vi "AlliGator Script Sum All Datasets in Folder.vi"(4 "Index Offsets (Default: None)":i32[](array[numeric]), 6 "Weights (Default: None)":dbl[](array[numeric]), 7 "Single File? (Default: False)":bool, 8 "Error In":errorcluster, 9 "AlliGator Data Series Type":T1, 10 "Path":path, 11 "Alligator Queue Elements in":T2[](array[typedef])) -> (0 "Error Out":errorcluster, 1 "Message":string, 2 "[Time-Series Path]":path[](array[path]), 3 "Alligator Queue Elements out":T2[](array[typedef]))   [LabVIEW 2021, in "AlliGator Accumulated Dataset.lvlib"]
doc: "Launches a series of steps loading each dataset in a series (including background correction) and adding them to a reset accumulated dataset. This script is followed by the usual series of steps after a new dataset is loaded (display, phasor plot update, phasor ratio or map overlay in image source and/or image ROI highlight in phasor plot)."
uses:
  AlliGator Accumulated Dataset.lvlib
  AlliGator Q Element.ctl
  AlliGator Q Event.ctl
  AlliGator Data Series Type.ctl
  AlliGator Variables List.ctl
  Alligator Elements Order in Action Stack.ctl
  AlliGator Settings List.ctl
  AlliGator Gate Arithmetic.ctl
  AlliGator Channel Arithmetic Action Parameters.ctl
  AlliGator Load Dataset Options.ctl
  AlliGator FLI Dataset Type.ctl
  AlliGator Add Action Array to Stack.vi
  <vilib>/Utility/error.llb/Error Cluster From Error Code.vi
  AlliGator Add Single Action to Stack.vi
  <vilib>/ErrorRing/Error Ring.xnode
  AlliGator Action Engine.lvlib
  AlliGator Globals, Variables & Constants.lvlib
  Strings/Strings.lvlib
  Files/Files.lvlib
  AlliGator Files.lvlib
  AlliGator Settings.lvlib
  AlliGator Dual-Channel Datasets.lvlib
panel:
  out "File Names":string[](array[string])
  out "# Time Points":i32
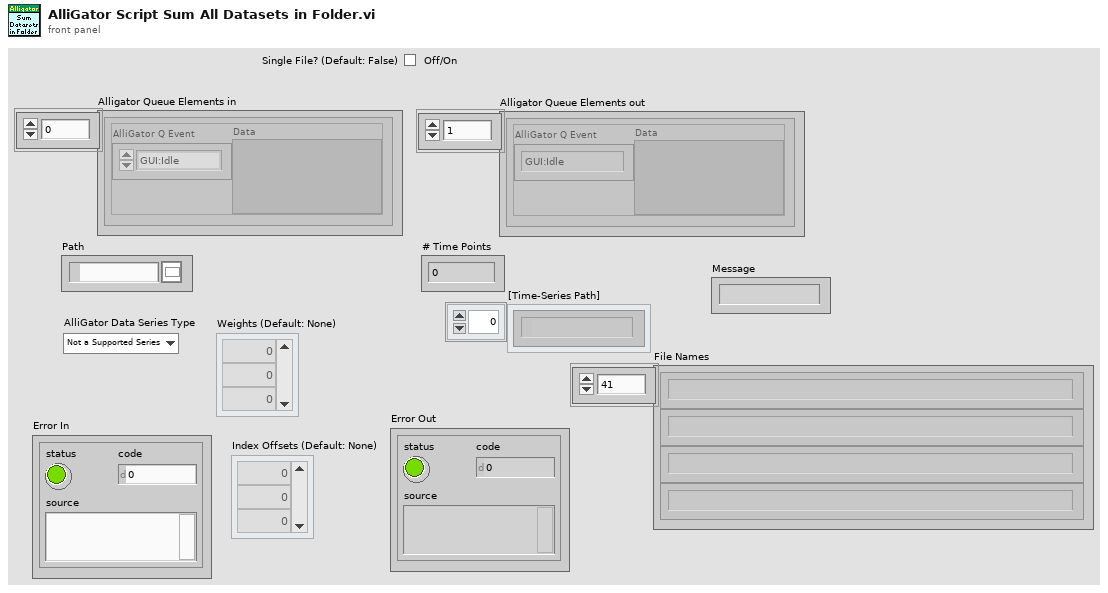
[diagram p1: front panel]
types:
  T1 = typedef "AlliGator Files.lvlib/AlliGator Data Series Type.ctl" = enum16{"Not a Supported Series", "Gate Images Folder Series", "SwissSPAD 2 Dataset Series", "B&H FLI Dataset Series", "PicoQuant PTU FLI Dataset Series", "PicoQuant BIN FLI Dataset Series", "Piccolo hist BIN FLI Dataset Series", "HDF5 FLI Dataset Series"}
  T2 = typedef "AlliGator Action Engine.lvlib/AlliGator Q Element.ctl" = cluster{"AlliGator Q Event":T3, "Data":variant}
  T3 = typedef "AlliGator Action Engine.lvlib/AlliGator Q Event.ctl" = enum16{"---- Files ----", "Files:Set Batch Export Files To Save", "Files:Set Dataset Loading & Pre-processing Options", "Files:Check #Frames in Dataset", "Files:Increment Frame Index", "Files:Open Mask Image", "Files:Open White Light Image", "Files:Open Single Dataset", "Files:New Folder of Folders Selected", "Files:Load File (all Types)_Scriptable", "Files:Move Flattened Series to Folders Series", "Files:Select Folder", "Files:Load FLI Dataset", "Files:Load Swiss SPAD 1 Dataset", "Files:Load Swiss SPAD 2 Dataset", "Files:Load .sdt FLI Dataset", "Files:Load .ptu FLI Dataset", "Files:Load .bin FLI Dataset", "Files:Load Single Gate Image Folder", "Files:Load I/m/phi Dataset (deprecated)", "Files:Load Single Image", "Files:Subtract Background File", "Files:Export FLI Dataset", "Files:Load HDF5 FLI Dataset", "Files:Set Destination File Path", "Files:Save Mask Image", "Files:Batch Conversion", "Files:New Folder Selected", "Files:Close FLI Dataset", "Files:Close FLI Dataset Series", "Files:Close White Light Image", "Files:Close Mask Image", "---- FLI Dataset ----", "FLI Dataset:Channel Arithmetic", "FLI Dataset:Export Average Lifetime Map as ASCII", "FLI Dataset:Export User-Defined Quantity Map as ASCII", "FLI Dataset:Python Function FLI Dataset Event", "FLI Dataset:ROI Analysis", "FLI Dataset:Tilted Logistic Square Gated IRF Characteristics Map", "FLI Dataset:Logistic Square Gated IRF Characteristics Map", "FLI Dataset:Square Gated IRF Characteristics Map", "FLI Dataset:Multi-ROI Single-Pixel Phasor Analysis", "FLI Dataset:Multi-ROI Single-Pixel NLSF Analysis", "FLI Dataset:All ROIs IRF Extraction", "FLI Dataset:All ROIs Decay Fit Non-Interactive (Fast + Individual IRF)", "FLI Dataset:All ROIs Phasor Analysis", "FLI Dataset:All ROIs Decay Fit", "FLI Dataset:Fluorescence Decay Statistics", "FLI Dataset:Update Decay Statistics Graph", "FLI Dataset:Get Decay from ROI", "FLI Dataset:All ROIs Average Lifetimes", "---- FLI Dataset Series ----", "FLI Dataset Series:Sum All Datasets in Series", "FLI Dataset Series:Add Dataset to Accumulated Dataset", "FLI Dataset Series:Display Accumulated Dataset", "FLI Dataset Series:Clear Dataset Series Sum", "FLI Dataset Series:Time-Series Analysis (NLSF)", "FLI Dataset Series:Time-Series Analysis (Phasor)", "---- Image ----", "Image:Update Image Profile Plots", "Image:Image Histogram Cursor Move", "Image:Image Histogram", "Image:Image Contrast", "Image:Set Image Histogram Cursor Move Flag", "Image:Clear Image Overlay", "Image:Use ROI as Search Area", "Image:Set ROI Diameter", "Image:Save Image Data as TIFF", "Image:Save Displayed Image with Overlay", "Image:Save Image Overlay Only", "Image:Save Image as Hot Pixel Mask", "Image:Change Source Image Color Palette", "Image:Copy Image to Clipboard", "Image:Source Image ROI Selection", "Image:Delete All ROIs", "Image:Delete All Unselected ROIs", "Image:Delete ROI", "Image:Merge All ROIs", "Image:Store ROI", "Image:Source Image ROI Storage", "Image:Export ROI Description to Notebook", "Image:Save ROI", "Image:Load ROI", "Image:Paste ROI Definition", "Image:Clear ROI", "Image:Identify ROIs in Mask Image", "Image:Create Complementary ROI", "Image:Create Contour ROI", "Image:Create ROI(s) from Pixels with Peak above Min_Scriptable", "Image:Create ROI(s) from Pixels with Intensity above Min_Scriptable", "Image:Compute ROI Statistics", "Image:Delete ROI(s) based on ROI Characteristics", "Image:Create ROI Grid", "Image:ROI to Individual Pixel ROIs", "Image:Python Function Source Image Event", "Image:Show Phasor Calibration Map ROI Centers", "Image:Convert ROI to Mask Image", "Image:Mouse Move", "Image:Mouse Up", "Image:Set Source Image Mouse Move Flag", "Image:Add Scale Bar Overlay", "Image:Delete Existing ROIs Option", "---- Decay ----", "Decay:Clear IRF/Reference Plot", "Decay:Clear Local IRFs", "Decay:Add Decay to Graph", "Decay:Smoothen Plot", "Decay:Smoothen Plot Tail", "Decay:Average Selected Plots", "Decay:Extract IRF", "Decay:Optimal IRF Extraction", "Decay:Threshold IRF", "Decay:Fit to Model IRF", "Decay:Fit IRF to Square Gate", "Decay:Fit IRF to Logistic Square Gate", "Decay:Fit IRF to Tilted Logistic Square Gate", "Decay:Create Bounding Cursors Set", "Decay:Export Bounding Cursors Definition to Notebook", "Decay:Denoise Plot", "Decay:Compute Cumulative Function", "Decay:Use as Reference Decay", "Decay:Show Reference Decay/IRF", "Decay:Extrapolate Decay", "Decay:Create Head & Tail Bounding Cursors", "Decay:Store Cursor-defined Head & Tail Fractions", "Decay:Rebin Plot", "Decay:1-Normalize Decay", "Decay:[0-1]-Normalize Plot", "Decay:Straighten Decay", "Decay:Shift Decay", "Decay:Fold Decay", "Decay:Fit Decay", "Decay:Global Fit of Selected Decays", "Decay:Post Global Fit Script", "Decay:Add Global Fit Parameters to Graph", "Decay:Add Decay Parameter(s) to Plot (Graph)", "Decay:Export Decay to Phasor Graph", "Decay:Plot Decay Shifts", "Decay:Compute Average Lifetime", "Decay:Plot Convolution", "Decay:Graph Tip Strip Update", "---- Decay Statistics ----", "Decay Statistics:Tip Strip Update", "---- Intensity Time Trace ----", "Intensity Time Trace:Use File Timestamp", "Intensity Time Trace:Load Intensity Corrections File", "Intensity Time Trace:Clear Intensity Corrections File", "Intensity Time Trace:Tip Strip Update", "---- Phasor Plot ----", "Phasor Plot:Build Phasor Plot", "Phasor Plot:Change Phasor Plot Color Palette", "Phasor Plot:Adjust Phasor Plot Display Range", "Phasor Plot:Highlight Image ROI in Phasor Plot", "Phasor Plot:Save Phasor Plot Image with Overlay", "Phasor Plot:Export Complex Phasor Map", "Phasor Plot:Export Phasor Ratio Map", "Phasor Plot:Export Average Lifetime Map", "Phasor Plot:Compute Phase Lifetime Histogram", "Phasor Plot:Compute Phasor Ratio Histogram", "Phasor Plot:Compute Phase Lifetime vs Intensity Scatter Plot", "Phasor Plot:Weber 2-Component Decomposition", "Phasor Plot:Update Phasor Color Map Vertices", "Phasor Plot:Clear Phasor Overlay", "Phasor Plot:Use Segment Extremities as References", "Phasor Plot:Use UC/Segment Intersections as References", "Phasor Plot:Use UC/Principal Axis Intersections as References", "Phasor Plot:Use UC/Linear Fit Intersections as References", "Phasor Plot:Update Phasor Plot Reference", "Phasor Plot:Show Local Phasor Info in Phasor Plot", "Phasor Plot:Update Phasor Plot State", "Phasor Plot:Phasor Plot ROI Storage", "Phasor Plot:Phasor Plot ROI Selection", "Phasor Plot:Python Function Phasor Plot Event", "Phasor Plot:Overlay Phasor ROI, Ratio or Map in Source Image", "Phasor Plot:Compute Decay of Selected Phasors", "Phasor Plot:Phasor at Image Pixel", "Phasor Plot:Mouse Move", "Phasor Plot:Mouse Up", "Phasor Plot:Display Range Mouse Move", "Phasor Plot:Set Mouse Move Flag", "---- Phasor Graph ----", "Phasor Graph:Calibrated Phasor Map Series", "Phasor Graph:Whole Image Phasor Scatter Plot (Todo)", "Phasor Graph:Get Phasor Value", "Phasor Graph:Create New Phasor Plot Dialog", "Phasor Graph:Update Last Phasor Value", "Phasor Graph:Update Phasor (m, phi)", "Phasor Graph:Remove Single Phasor from Plot", "Phasor Graph:Add Single Phasor to Plot", "Phasor Graph:Remove Phasor Plot", "Phasor Graph:Remove Selected Phasor Plots", "Phasor Graph:Clear Phasor Data", "Phasor Graph:Clear Phasor Graph", "Phasor Graph:Cursor Move", "Phasor Graph:Draw Cursor Connecting Line", "Phasor Graph:Clear Cursor Connecting Line", "Phasor Graph:Find UC Intersection", "Phasor Graph:Use UC/Cursor-Defined Line Intersections", "Phasor Graph:Use Selected Plots Fitted Line/UC Intersections", "Phasor Graph:Use Selected Plots Principal Axis/UC Intersections", "Phasor Graph:Show Single Phasor", "Phasor Graph:Save Single Phasor Plot", "Phasor Graph:Save All Phasor Plots", "Phasor Graph:Load Phasor Plot(s)", "Phasor Graph:Phasor Multiplication", "Phasor Graph:Compute Average Phasor", "Phasor Graph:Compute Multiple Average Phasors (Selected Plots)", "Phasor Graph:Export Single Phasor Plot Phase Lifetimes", "Phasor Graph:Phase Lifetime Trajectory", "Phasor Graph:Phase Lifetime vs Intensity Scatter Plot (deprecated)", "Phasor Graph:Parameter 2 vs Parameter 1 Scatter Plot", "Phasor Graph:Use Cursor n Location", "Phasor Graph:Set Reference n to Current Phase Lifetime Value", "Phasor Graph:Set Reference n to Lifetime Value", "Phasor Graph:Set Cursor n Location", "Phasor Graph:Save Phasor Graph Image", "Phasor Graph:Update SEPL Plot", "Phasor Graph:Export Single Phasor Plot Data", "Phasor Graph:Export Selected Phasor Plots Data", "Phasor Graph:Python Function Phasor Graph Event", "Phasor Graph:Tip Strip Update", "---- Calibration ----", "Calibration:Set Calibration Type", "Calibration:Load/Save Phasor Calibration", "Calibration:Load/Save Phasor Calibration Series", "Calibration:Load/Save Phasor Calibration Map", "Calibration:Use as Calibration", "Calibration:Compute Optimal Calibration from Phasor References", "Calibration:Clear Phasor Calibration", "Calibration:Use as Calibration Series", "Calibration:Use as Calibration Map", "Calibration:Clear Calibration Series", "Calibration:Clear Calibration Map", "Calibration:Apply Phasor Calibration", "Calibration:Update Single Plot Calibration", "Calibration:Update Multiple Plots Calibration", "Calibration:Clear Single Plot Calibration", "Calibration:Clear All Plots Calibrations", "Calibration:Clear Plot(s) Calibration(s)?", "Calibration:Phasor Calibration Maps (# Gates Series)", "---- Phasor Ratio ----", "Phasor Ratio:Clear Reference n", "Phasor Ratio:Toggle Selected Plot(s)  Lock to Reference 1", "Phasor Ratio:Use as Reference n", "Phasor Ratio:Send Reference n to Notebook", "Phasor Ratio:Toggle Selected Plot(s)  Lock to Reference 2", "Phasor Ratio:Compute Phasor Ratio at Mouse Location", "Phasor Ratio:Compute Phasor Plot's Average Phasor Ratio", "Phasor Ratio:Compute Time-Series Phasor Ratios", "Phasor Ratio:Fit Line to Phasor Ratio Plot", "Phasor Ratio:Save References", "Phasor Ratio:Load References", "Phasor Ratio:Update Phasor Reference 1", "Phasor Ratio:Update Phasor Reference 2", "Phasor Ratio:Move Cursor n to Reference n", "Phasor Ratio:Use as Phasor Reference 1 Lifetime", "Phasor Ratio:Use as Phasor Reference 2 Lifetime", "Phasor Ratio:Export Phasor Ratio Map as ASCII", "Phasor Ratio:Tip Strip Update", "---- Lifetime & Other Parameters Graph ----", "Lifetime:Tip Strip Update", "---- Decay Fit Parameter Map ----", "Decay Fit Parameter Map:Export ROI NLSF Data as ASCII", "Decay Fit Parameter Map:Set Decay Fit  Parameter Map Selection", "Decay Fit Parameter Map:Build Decay Fit Parameter Map", "Decay Fit Parameter Map:Change Decay Fit Parameter Map Color Palette", "Decay Fit Parameter Map:Export Decay Fit Parameter Map Data as ASCII", "Decay Fit Parameter Map:Export All Decay Fit Parameter Maps Data as ASCII", "Decay Fit Parameter Map:Send Map Data to Lifetime Graph", "Decay Fit Parameter Map:Save Decay Fit Parameter Map Image", "Decay Fit Parameter Map:Save-Load IRFs & Fit Data", "Decay Fit Parameter Map:Update Local Decay Plots", "Decay Fit Parameter Map:Python Function Decay Fit Parameters Map Event", "Decay Fit Parameter Map:Overlay Decay Fit Parameter Map in Source Image", "Decay Fit Parameter Map:Plot Map Data vs Intensity", "Decay Fit Parameter Map:Mouse Up", "Decay Fit Parameter Map:Display Range Mouse Move", "---- Generic Graph ----", "Generic Graph:Generic XY Graph Event", "Generic Graph:Python Function XY Graph Event", "Generic Graph:New Plot", "Generic Graph:Save Plot", "Generic Graph:XY Plot Histogram", "Generic Graph:Set XY Graph Plot Name", "Generic Graph:Set Last Cursor Style", "Generic Graph:Tip Strip Update", "---- GUI ----", "GUI:Start Script", "GUI:Type of Displayed Image Changed", "GUI:Gate Image Slide Changed", "GUI:Show Busy Icon", "GUI:Show Busy Icon & Abort Button", "GUI:Hide Busy Icon", "GUI:Hide Busy Icon & Abort Button", "GUI:Abort", "GUI:End Script", "GUI:Start Timing", "GUI:End Timing", "GUI:Set State Indicator", "GUI:Send Parameters JSON Strings to Clipboard", "GUI:Set Gate Step", "GUI:Idle", "GUI:Initialization", "GUI:Quit", "GUI:Increment Dataset Index", "GUI:Set Dataset Index to -1", "GUI:Time Series Slider Moved", "GUI:Time Series Slider Changed", "GUI:Toggle Playback or Loop", "GUI:Playback Script", "GUI:Set Phasor Frequency", "GUI:Open Window", "DEBUG"}
  T4 = typedef "AlliGator Globals, Variables & Constants.lvlib/AlliGator Variables List.ctl" = enum16{"---- GUI ----", "Initialization Status", "State Indicators Refnum", "Original AlliGator Menu Items", "Current Action Loop State", "Script in progress", "Playback", "Loop Playback", "Search ROI Used", "Search ROI", "Decay Graph Max Legend Size", "Intensity Graph Max Legend Size", "Decay Statistics Graph Max Legend Size", "Phasor Graph Max Legend Size", "Phasor Ratio Graph Max Legend Size", "Lifetime Graph Max Legend Size", "---- Files ----", "Export Dataset Frames as Individual Files", "Show Batch Export Help Balloons", "Frames in Dataset", "ptu File Frame Start Indices", "Current Frame in Dataset", "Current Frame Timestamp", "------ Python Plugins ------", "Python Plugins Information", "Python Session", "Valid Python Session?", "---- Source Image ----", "Dataset Loaded", "Dataset Metadata", "Dataset Channel", "Dataset Data Description", "Background Dataset Metadata", "Background Dataset Channel", "Background Dataset Data Description", "Background File Subtraction", "Background File Path", "Background File Pile-up Correction", "Background File Pixel Well Capacity", "Background File Scaling Factor", "Source Image ROIs", "Current Source Image ROI", "Source Image ROI Event Refnum", "X_Source Image Display Range", "X_Source Image Palette Information", "Source Image Palette List", "Source Image Scale", "Current Dataset Load Settings", "Source Image:ROI Overlay Color", "---- Image Profile Window ----", "Image Profile:Overlay ROI in Source Image", "Image Profile Window Event Refnum", "Image Profile:IntensityType", "Image Profile:Intensity Average Type", "Image Profile:Intensity-weighted SDV", "Image Profile:Box Profile Type", "Image Profile Window Open", "Image Profile:Plotted Fit Parameter", "X_Type of Displayed Image", "X_Time Gate Slider", "Dataset Path", "Source Image Overlay to Erase", "Is Displayed Image Accumulated", "White Light Image Modified", "Mask Image Modified", "Macrotime Gate Separation", "------ Phasor Graph -------", "Phasor Graph:Show Line", "---- Phasor Plot ---", "Phasor Plot Parameters Changed", "FLI Dataset Modified since last Phasor Plot Calculation", "Phasor Harmonics Data", "Selected Phasor Harmonics", "Phasor Harmonic Manager Event Refnum", "Phasor Plot ROIs", "Current Phasor Plot ROI", "Phasor Plot ROI Event Refnum", "Phasor Plot Image Reference Points", "Phasor Plot Computed", "Phasor Plot Palette Information", "Phasor Plot Palette List", "Phasor Ratio Palette Information", "Phasor Ratio Palette List", "Phasor Image Scale", "Phasor Plot Image Overlay to Erase", "Phasor Plot Image Elements to Update", "Current Phasor Plot Calculation Parameters", "Current Phasor Calibration Options", "Reset Cumulated Phasor Plot", "Phasor Ratio Reference 1", "Phasor Ratio Lifetime Reference 1", "Phasor Ratio Reference 1 Frequency", "Phasor Ratio Reference 2", "Phasor Ratio Lifetime Reference 2", "Phasor Ratio Reference 2 Frequency", "---- Decay Analysis ----", "Number of Selected Decays to Fit", "LS Fit Results", "LAR Fit Results", "BS Fit Results", "Last Decay Max - Min", "Best Fit Parameters", "Best Fit Parameter Names", "Actual Size X", "Actual Size Y", "Binning X", "Binning Y", "Actual # Gates", "Dataset Number", "Gates to...", "Gates Skipped", "Gates to keep", "Gate Step", "Gate Separation", "Reversed Gates", "Pile-up Correction", "Pixel Well Capacity", "Background Subtracted", "Background Subtraction Method", "Background Definition Range", "Background File (deprecated)", "Number of Dataset Accumulated", "Array of Accumulated Dataset Paths", "Do Averaged Datasets", "Destination File Path", "Process Plot Target", "Use 1/D as Phasor Frequency", "---- Decay Fit Parameter Map -----", "Decay Fit Parameter Map Palette Information", "Decay Fit Parameter Map Palette List", "Local Decay Graph Window Event Refnum", "------- Local Decay Window ---------", "Use normalized IRF for convolution", "----- Miscellaneous ----", "Skippable Dialog Windows Status"}
  T5 = enum16{"Start Script", "Load & Analyze Data", "End Script"}
  T6 = typedef "AlliGator Action Engine.lvlib/Alligator Elements Order in Action Stack.ctl" = enum16{"Enqueue 2 AFTER 1", "Enqueue 2 BEFORE 1"}
  T7 = typedef "AlliGator Dual-Channel Datasets.lvlib/AlliGator Channel Arithmetic Action Parameters.ctl" = cluster{"Channel Name":u16, "Channel Arithmetic":T8}
  T8 = typedef "AlliGator Settings.lvlib/AlliGator Gate Arithmetic.ctl" = enum16{"None", "INT-G2", "G2/INT*<INT>", "(1 - G2/INT)*<INT>"}
  T9 = typedef "AlliGator Settings.lvlib/AlliGator Settings List.ctl" = enum16{"GUI:Visible Settings Tab", "GUI:Last Run Version", "Source Image:Use Image Histogram for Contrast", "Source Image:Low Count Pixels Rejection Options", "Source Image:High Count Pixels Rejection Options", "Source Image:Use Image Brightness", "Source Image:Blend Overlay with Image Background", "Source Image:Use Fixed ROI Diameter", "Source Image:ROI Diameter", "Source Image:ROI Center Color", "Source Image:Peak Threshold", "Source Image:Intensity Threshold", "Source Image:Image Binning Options", "Source Image:Image Smoothing Options", "Source Image:Image Histogram Active", "Source Image:Invert Binary Mask", "Source Image:Hot Pixel Removal", "Source Image:Overlay Analyzed ROI Center", "Source Image:Auto-Adjust Contrast", "Source Image:Histogram Lower Percentile", "Source Image:Histogram Upper Percentile", "Source Image:Save Source Image", "Source Image:Scale Bar Options", "Source Image:Image Resolution (Pixel Size)", "Source Image:Flatfield Correction", "Data Information:Gate Width", "Data Information:Nanotime Gate Separation", "Data Information:Macrotime Gate Separation", "Data Information:Gate Step", "Data Information:# Gates", "Data Information:Gate Image Exposure", "Data Information:Gate Image Integration", "Data Information:Gates to Skip", "Data Information:Gates to Keep", "Data Information:Define Gates to", "Data Information:Channel Name", "Data Information:Available Channel Names", "Data Information:Channel Arithmetic", "Data Information:Background File Subtraction", "Data Information:Background File", "Data Information:Background Scaling Factor", "Data Information:Background Pile-up Correction", "Data Information:Background Pixel Well Capacity", "Data Information:Laser Period", "Data Information:SYNC Period", "Data Information:Pile-up Correction", "Data Information:Pixel Well Capacity", "Data Information:Dataset Scaling Factor", "Fluorescence Decay_Decay Pre-Processing:Reverse Gates", "Fluorescence Decay_Decay Pre-Processing:Verbose Decay Pre-Processing", "Fluorescence Decay_Decay Pre-Processing:Use Decay Pre-Processing", "Fluorescence Decay_Decay Pre-Processing:Background Subtraction", "Fluorescence Decay_Decay Pre-Processing:Background Definition Range", "Fluorescence Decay_Decay Pre-Processing:Baseline Subtraction Method", "Fluorescence Decay_Decay Pre-Processing:Operations Order", "Fluorescence Decay_Decay Pre-Processing:Smoothing Parameter", "Fluorescence Decay_Decay Pre-Processing:Shift Decay", "Fluorescence Decay_Decay Pre-Processing:Decay Shift Parameters", "Fluorescence Decay_Decay Pre-Processing:Fold Decay", "Fluorescence Decay_Decay Pre-Processing:# Folds", "Fluorescence Decay_Decay Pre-Processing:1-Normalize Decay", "Fluorescence Decay_Decay Pre-Processing:[0-1]-Normalize Decay", "Fluorescence Decay_Decay Pre-Processing:Smoothen Decay", "Fluorescence Decay_Decay Pre-Processing:Extrapolate Decay", "Fluorescence Decay_Decay Pre-Processing:Use Periodicity", "Fluorescence Decay_Decay Pre-Processing:Use Cursors", "Fluorescence Decay_Decay Pre-Processing:Tail Fraction", "Fluorescence Decay_Decay Pre-Processing:Head Fraction", "Fluorescence Decay_Decay Pre-Processing:Additional Points", "Fluorescence Decay_Decay Pre-Processing:Straighten Decay", "Fluorescence Decay_Decay Pre-Processing:Constant Background", "Fluorescence Decay_Decay Pre-Processing:Pixel-Normalize Decay", "Fluorescence Decay_Advanced Analysis:Extract IRF instead of Decay", "Fluorescence Decay_Advanced Analysis:IRF Extraction Options", "Fluorescence Decay_Advanced Analysis:IRF Optimization Options", "Fluorescence Decay_Advanced Analysis:Square Pulse Options", "Fluorescence Decay_Advanced Analysis:IRF Order", "Fluorescence Decay_Advanced Analysis:IRF Time Constants", "Fluorescence Decay_Advanced Analysis:Wavelet Analysis Options", "Fluorescence Decay_Advanced Analysis:Average Lifetime Options", "Fluorescence Decay_Fit Options:Fit Options", "Fluorescence Decay_Fit Options:Use Legacy Fitting Approach", "Fluorescence Decay_Fit Options:Use Data Information Laser Period", "Fluorescence Decay_Fit Parameters:Displayed Fit Parameters", "Fluorescence Decay_Fit Parameters:Fit Parameter Constraints", "Fluorescence Decay_Fit Parameters:Export Tabulated Results", "Fluorescence Decay_Fit Parameters:MLE Baseline Offset Type", "Fluorescence Decay_Fit Parameters:MLE Baseline Offset", "Fluorescence Decay_Fit Parameters:Guess Parameter Names", "Fluorescence Decay_Fit Parameters:Guess Parameter Values", "Fluorescence Decay_Fit Parameters:Guess Parameters Options", "Fluorescence Decay_Styles:Show Last Decay Only", "Fluorescence Decay_Styles:Decay Graph Color Array", "Fluorescence Decay:Decay Graph Active", "Fluorescence Decay Statistics:Min Peak Value", "Fluorescence Decay Statistics:Reject Low Decay Peak Pixels", "Fluorescence Decay Statistics:Reject High Decay Peak Pixels", "Fluorescence Decay Statistics:Max Peak Value", "Time Traces:Use File Timestamp", "Time Traces:Time Step", "Time Traces:Use Intensity Correction File", "Time Traces:Intensity Correction File", "Phasor Plot:Phasor Plot Smoothing Options", "Phasor Plot:Phasor Plot Size", "Phasor Plot:Phasor Plot Graphics Options", "Phasor Plot:Cumulative Phasor Plot", "Phasor Plot:Use Phasor Brightness", "Phasor Plot:Blend Overlay with Phasor Background", "Phasor Plot:Save Phasor Plot", "Phasor Plot:Show References", "Phasor Plot:Phasor Ratio Decay Range", "Phasor Plot:Exponential Fading", "Phasor Plot:Phasor Ratio Reference Colors", "Phasor Plot:Reference Radius", "Phasor Plot:Show Color Map Vertices", "Phasor Plot:Phasor Plot Active", "Phasor Plot:Phasor Ratio Color Map Type", "Phasor Plot:Phasor Ratio Color Map", "Phasor Plot:Phasor Ratio Display Range", "Phasor Plot:Selected Image ROI(s)", "Phasor Plot:All Image ROIs", "Phasor Plot:Selected Phasor Plot ROI(s)", "Phasor Plot:All Phasor Plot ROIs", "Phasor Plot:Phasor Ratio Color-Coded Quantity", "Phasor Plot:Store Phasor Harmonics", "Phasor Plot:Draw Reference Segment", "Phasor Plot:User-Defined Quantity", "Phasor Graph:Phasor Frequency", "Phasor Graph:Phasor Ratio Type", "Phasor Graph:Pixel-level Phasor Computation", "Phasor Graph:Save Phasor Graph", "Phasor Graph:Phasor Graph Active", "Phasor Graph:Phasor SDV Options", "Phasor Calibration:Use Backup Calibration if needed", "Phasor Graph:Define Shortest Lifetime as", "Phasor Calibration:Backup Calibration Type", "Phasor Calibration:Calibration Type", "Phasor Calibration:Calibration Lifetime", "Phasor Calibration:Calibration Map Algorithm", "Single-Exponential Phasor Locus (SEPL):Gate Parameters", "Single-Exponential Phasor Locus (SEPL):User-defined Gate", "Single-Exponential Phasor Locus (SEPL):User-defined IRF", "Single-Exponential Phasor Locus (SEPL):Phasor Parameters", "Single-Exponential Phasor Locus (SEPL):Decay & IRF Parameters", "Single-Exponential Phasor Locus (SEPL):Display Parameters", "Lifetime Analysis:Decay Analysis Parameters", "Lifetime Analysis:Lifetime Map Active", "Plugins:Python Settings", "Miscellaneous:Verbose Mode", "Miscellaneous:Beep after Script", "Miscellaneous:Saved Image File Format", "Miscellaneous:Exported Gate Image Settings", "Miscellaneous:Include Loading in Timing", "Miscellaneous:Verbose Settings Mode", "Miscellaneous:Histogram Options", "Miscellaneous:Beep on Error", "Miscellaneous:# Logical Processors Used", "Miscellaneous:ROI Description Max Characters", "Miscellaneous:Verbose Error Mode", "Miscellaneous:Transparent Mask Color"}
  T10 = typedef "AlliGator Files.lvlib/AlliGator FLI Dataset Type.ctl" = enum16{"HDF5 FLI Dataset", "Gate Image Folder", ".sdt FLI Dataset (Becker & Hickl)", ".ptu FLI Dataset (PicoQuant)", "SS1 FLI Dataset", "SS2 FLI Dataset", "I/m/phi Dataset", ".bin FLI Dataset (PicoQuant Binned)", ".bin FLI Dataset (Piccolo Binned)"}
  T11 = typedef "AlliGator Files.lvlib/AlliGator Load Dataset Options.ctl" = cluster{"FLI Dataset Type":T10, "No Dialog?":bool, "File Path":path}
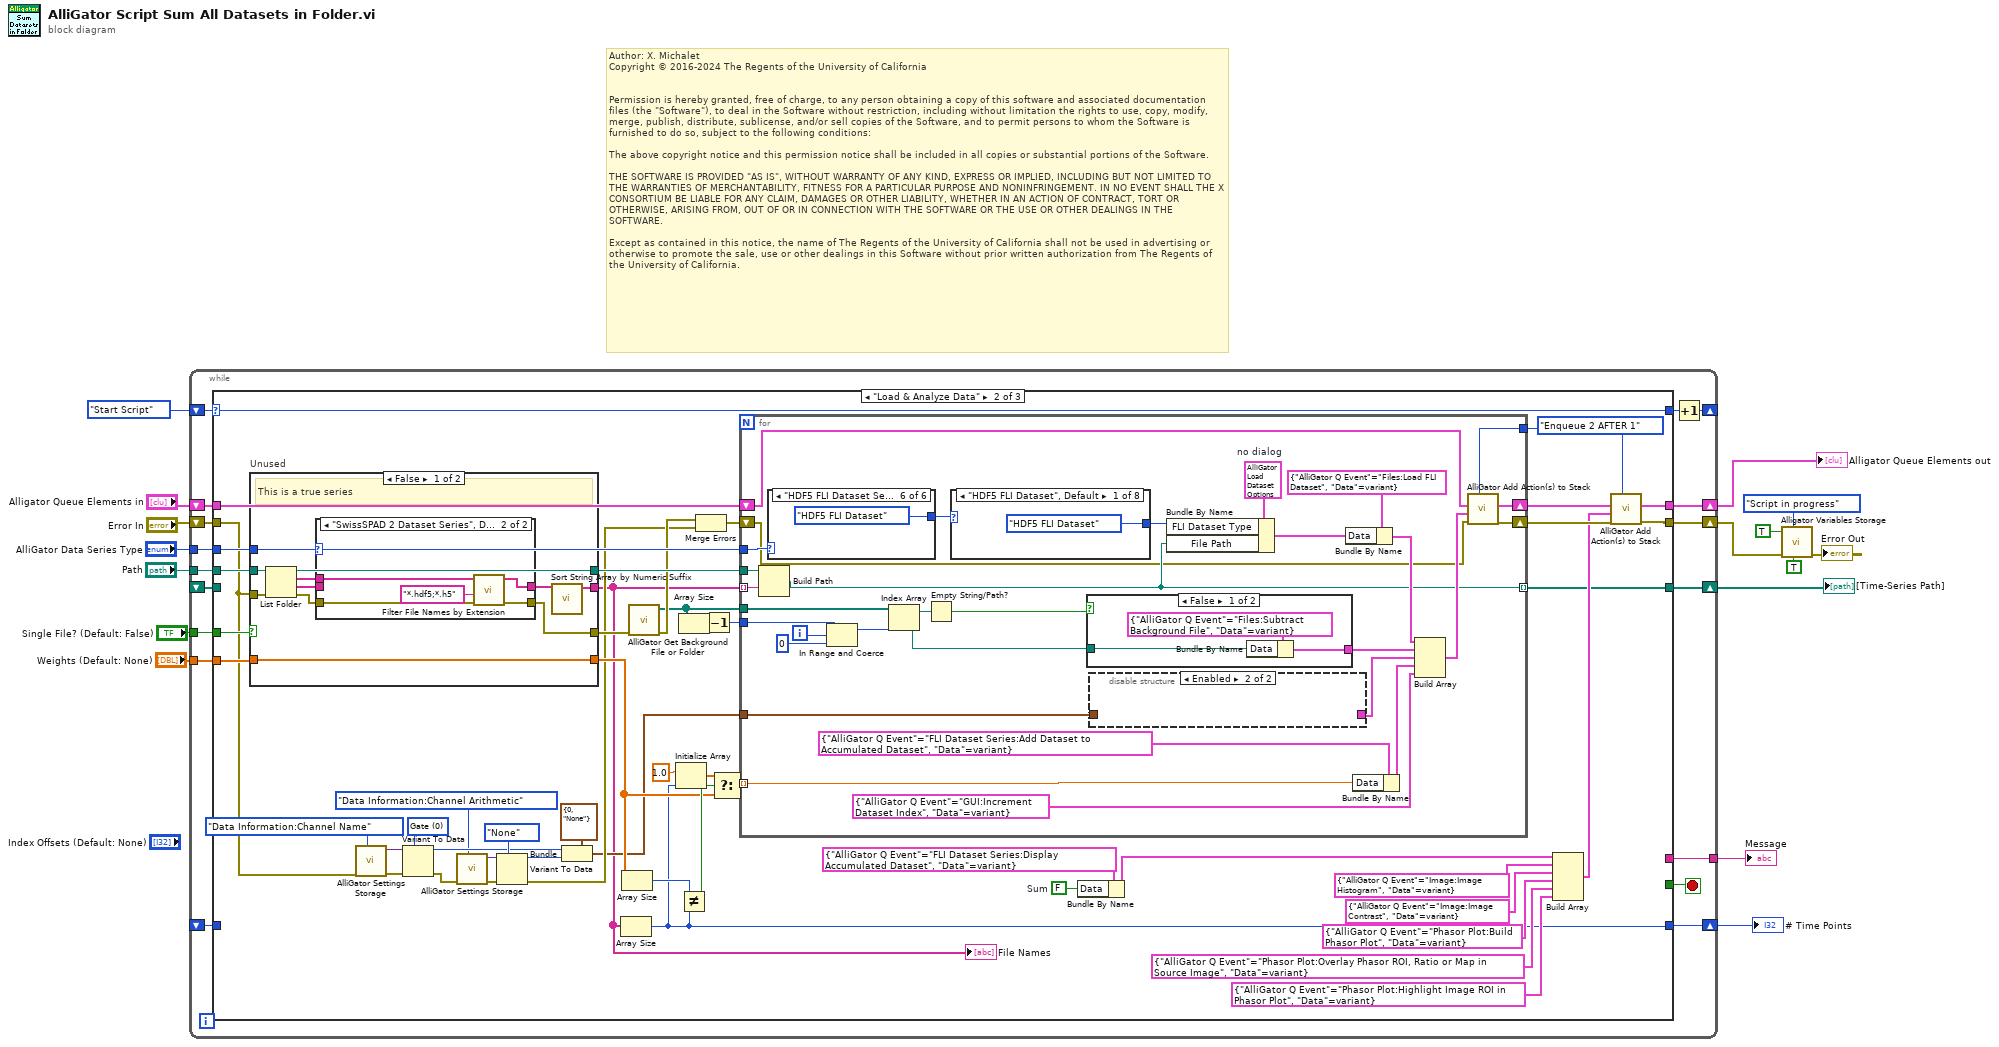
[diagram p0: block diagram]
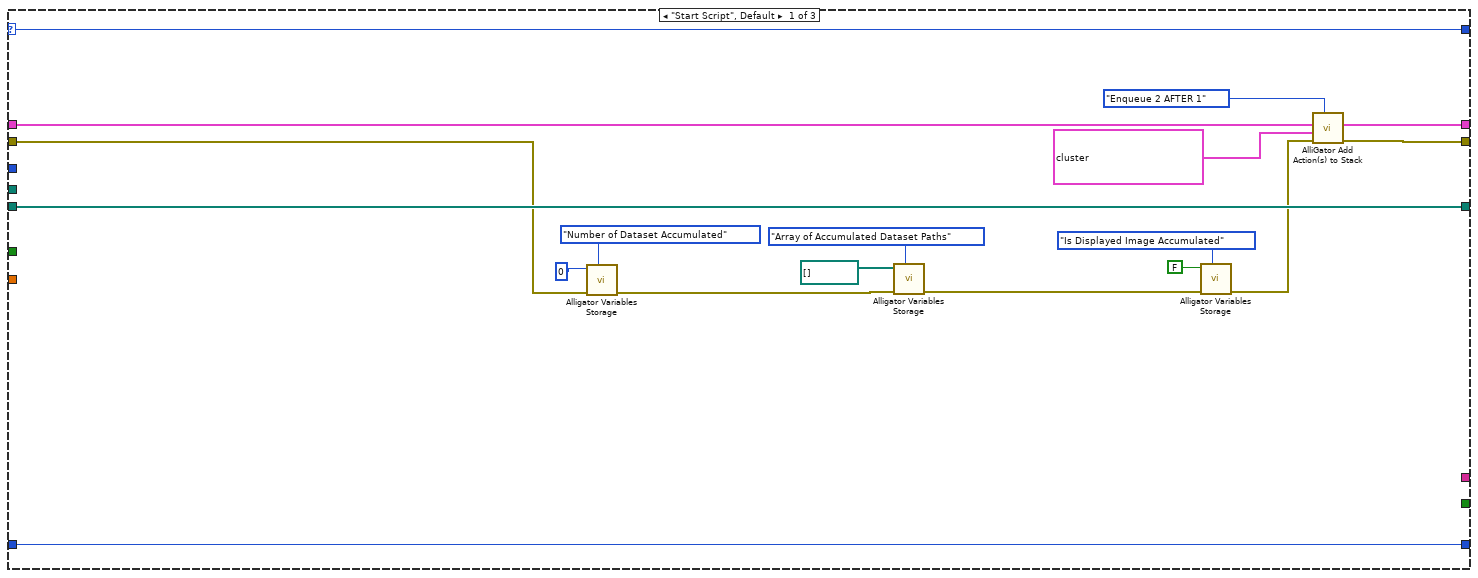
[diagram p2: hidden frame]
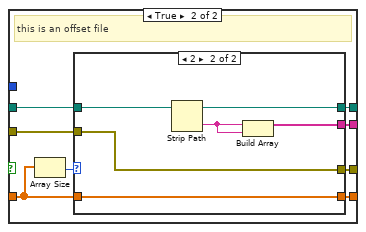
[diagram p4: hidden frame]
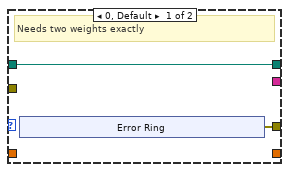
[diagram p5: hidden frame]
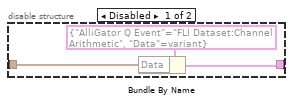
[diagram p6: hidden frame]
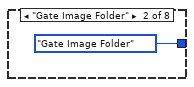
[diagram p7: hidden frame]
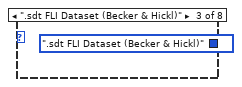
[diagram p8: hidden frame]
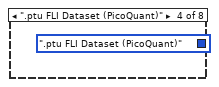
[diagram p9: hidden frame]
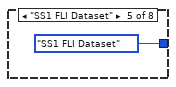
[diagram p10: hidden frame]
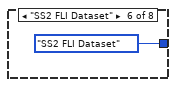
[diagram p11: hidden frame]
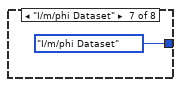
[diagram p12: hidden frame]
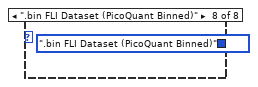
[diagram p13: hidden frame]
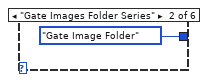
[diagram p16: hidden frame]
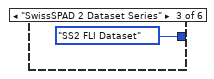
[diagram p17: hidden frame]
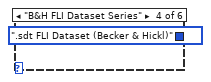
[diagram p18: hidden frame]
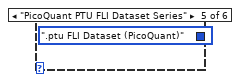
[diagram p19: hidden frame]
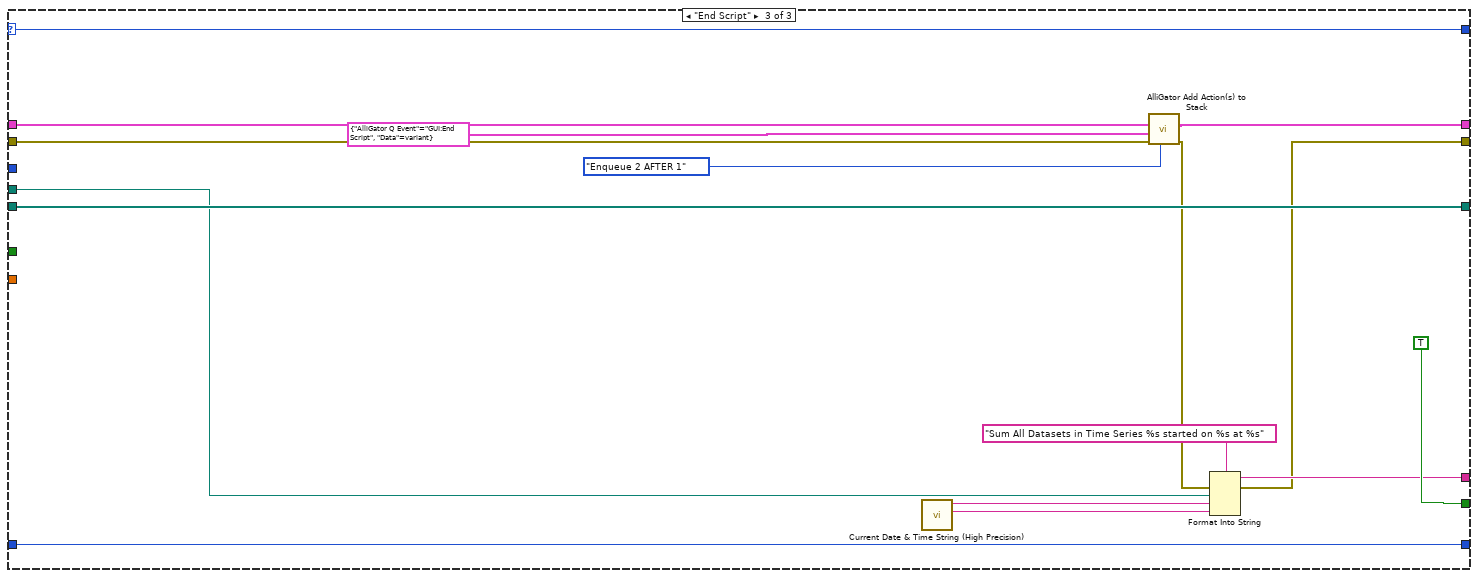
[diagram p20: hidden frame]
diagram:
  # "Author: X. Michalet\nCopyright © 2016-2024 The Regents of the University of California\n \n\nPermission is hereby granted, free of charge, to any person obtaining a copy of this software and associated documentation files (the \"Software\"), to deal in the Software without restriction, including without limitation the rights to use, copy, modify, merge, publish, distribute, sublicense, and/or sell copies of the Software, and to permit persons to whom the Software is furnished to do so, subject to the following conditions:\n\nThe above copyright notice and this permission notice shall be included in all copies or substantial portions of the Software.\n\nTHE SOFTWARE IS PROVIDED \"AS IS\", WITHOUT WARRANTY OF ANY KIND, EXPRESS OR IMPLIED, INCLUDING BUT NOT LIMITED TO THE WARRANTIES OF MERCHANTABILITY, FITNESS FOR A PARTICULAR PURPOSE AND NONINFRINGEMENT. IN NO EVENT SHALL THE X CONSORTIUM BE LIABLE FOR ANY CLAIM, DAMAGES OR OTHER LIABILITY, WHETHER IN AN ACTION OF CONTRACT, TORT OR OTHERWISE, ARISING FROM, OUT OF OR IN CONNECTION WITH THE SOFTWARE OR THE USE OR OTHER DEALINGS IN THE SOFTWARE.\n\nExcept as contained in this notice, the name of The Regents of the University of California shall not be used in advertising or otherwise to promote the sale, use or other dealings in this Software without prior written authorization from The Regents of the University of California."
  n1 = while {
    tunnel: "Path" -> [w32]
    shift-right: [w29] -> w11
    shift-left: "Error In" -> [w33]
    shift-right: [w27] -> _
    shift-left: T5."Start Script" -> [w30]
    shift-right: [w25] -> w12
    shift-left: "Alligator Queue Elements in" -> [w31]
    tunnel: "AlliGator Data Series Type" -> [w24]
    shift-right: [w22] -> w2
    shift-left: _ -> [w21]
    shift-right: [w23] -> w5
    shift-left: _ -> [w20]
    tunnel: "Weights (Default: None)" -> [w19]
    tunnel: "Single File? (Default: False)" -> [w18]
    tunnel: [w17] -> w1
    stop <- w26 stop-if-true
    n2 = case shown="\"Load & Analyze Data\"" w30 {
      selector: w30 -> [w51 w101 w204]
      tunnel: w33 -> [w46 w60 w201]
      tunnel: w32 -> [_ w100 w193]
      tunnel: w31 -> [w43 w102 w202]
      tunnel: [w38 w96 w190] -> w29
      tunnel: [w51 w101 w204] -> w28
      tunnel: [_ _ TRUE] -> w26
      tunnel: [w42 w98 w199] -> w25
      tunnel: w24 -> [_ w80 _]
      tunnel: [w49 w78 w195] -> w23
      tunnel: [w50 w74 w196] -> w22
      tunnel: w21 -> [w50 _ w196]
      tunnel: w20 -> [w49 _ w195]
      tunnel: w19 -> [_ w81 _]
      tunnel: w18 -> [_ w82 _]
      tunnel: [_ _ w192] -> w17
      frame "Start Script", Default {
        n3 = call "Alligator Variables Storage.vi"("AlliGator Variable"=AlliGator_Variables_List."Number of Dataset Accumulated" ("Alligator Variable"), "Error In"=w46, "Data in"=0) -> ("Error Out"=w39:errorcluster)  [unwired: 6 in, 2 out]
        n4 = call "Alligator Variables Storage.vi"("AlliGator Variable"=AlliGator_Variables_List."Array of Accumulated Dataset Paths" ("Alligator Variable"), "Error In"=w39, "Data in"=path[] [] ("path out")) -> ("Error Out"=w36:errorcluster)  [unwired: 6 in, 2 out]
        n5 = call "Alligator Variables Storage.vi"("AlliGator Variable"=AlliGator_Variables_List."Is Displayed Image Accumulated" ("Alligator Variable"), "Error In"=w36, "Data in"=FALSE) -> ("Error Out"=w34:errorcluster)  [unwired: 6 in, 2 out]
        n6 = call-poly "AlliGator Add Action(s) to Stack.vi"("Elements Order in Action Stack (Default: 2 BEFORE 1)"=Alligator_Elements_Order_in_Action_Stack."Enqueue 2 AFTER 1", "Error In"=w34, "Alligator Queue Element 2"=T2[] [{"AlliGator Q Event"=enum."GUI:Start Script", "Data"=variant}, {"AlliGator Q Event"=enum."GUI:Set Dataset Index to -1", "Data"=variant}] ("Alligator Atomic Action"), "Alligator Queue Element 1"=w43) -> ("Error Out"=w38:errorcluster, "Alligator Queue Element 1 (+ 2)"=w42:T2[])  [unwired: 6 in]
      }
      frame "Load & Analyze Data" {
        w64 = u16 0 items=["Gate"] ("Gate Name")
        w76 = FALSE  # Sum
        w89 = Alligator_Elements_Order_in_Action_Stack."Enqueue 2 AFTER 1" ("Elements Order in Action Stack (Default: 2 BEFORE 1)")
        n7 = case "Unused" shown="False" w82 {
          tunnel: w60 -> [w113 w124]
          tunnel: [w103 w123] -> w73
          tunnel: w100 -> [w112 w128]
          tunnel: [w108 w127] -> w75
          tunnel: [w107 w126] -> w55
          tunnel: w81 -> [w105 w122]
          tunnel: w80 -> [w106 _]
          tunnel: [w105 w121] -> w79
          frame False {
            # "This is a true series"
            n8 = List Folder(path=w112, error in=w113) -> (path out=w108:path, filenames=w111:string[], folder names=w110:string[], error out=w104:errorcluster)  [unwired: 2 in]
            n9 = case shown="\"SwissSPAD 2 Dataset Series\", Default" w106 {
              tunnel: [w115 w119] -> w109
              tunnel: w111 -> [_ w120]
              tunnel: w110 -> [w115 _]
              tunnel: w104 -> [w114 w117]
              tunnel: [w114 w116] -> w103
              frame "Gate Images Folder Series" {
              }
              frame "SwissSPAD 2 Dataset Series", Default {
                n10 = call "Filter File Names by Extension.vi"("Error In"=w117, "patterns"="*.hdf5;*.h5", "filenames in"=w120) -> ("Error Out"=w116:errorcluster, "filenames out"=w119:string[])  [unwired: 6 in, 1 out]
              }
            }
            n11 = call "Sort String Array by Numeric Suffix.vi"("String Array"=w109) -> ("Sorted String Array"=w107:string[])  [unwired: 8 in, 2 out]
          }
          frame True {
            # "this is an offset file"
            n12 = Array Size(array=w122) -> (size(s)=w125:i32)
            n13 = case shown="2" w125 {
              tunnel: w128 -> [w130 w140]
              tunnel: [w130 w139] -> w127
              tunnel: [_ w138] -> w126
              tunnel: w124 -> [_ w136]
              tunnel: [w129 w136] -> w123
              tunnel: w122 -> [_ w135]
              tunnel: [_ w135] -> w121
              frame 0, Default {
                # "Needs two weights exactly"
                n14 = xnode "Error Ring"() -> ("error out"=w129:errorcluster)
              }
              frame 2 {
                n15 = Strip Path(path=w140) -> (stripped path=w139:path, name=w137:string)
                n16 = Build Array(w137, w137) -> (w138:string[])
              }
            }
          }
        }
        "File Names" <- w55
        n17 = call "AlliGator Settings Storage.vi"("AlliGator Settings List"=AlliGator_Settings_List."Data Information:Channel Name", "Error In"=w60) -> ("Error Out"=w65:errorcluster, "Variant Data out"=w67:variant)  [unwired: 8 in]
        n18 = Variant To Data(error in=w65, type=w64, Variant=w67) -> (data=w63:u16, error out=w61:errorcluster)
        n19 = call "AlliGator Settings Storage.vi"("AlliGator Settings List"=AlliGator_Settings_List."Data Information:Channel Arithmetic", "Error In"=w61) -> ("Error Out"=w70:errorcluster, "Variant Data out"=w71:variant)  [unwired: 8 in]
        n20 = Variant To Data(error in=w70, type=AlliGator_Gate_Arithmetic."None" ("Gate Arithmetic"), Variant=w71) -> (data=w68:T8, error out=w57:errorcluster)
        n21 = Bundle(cluster=T7 {"Channel Name"=0, "Channel Arithmetic"=enum."None"} ("output cluster"), "Channel Name"=w63, "Channel Arithmetic"=w68) -> (w56:T7)
        n22 = Array Size(array=w55) -> (size(s)=w78:i32)
        n23 = Array Size(array=w79) -> (size(s)=w85:i32)
        n24 = call "AlliGator Get Background File or Folder.vi"("Error In"=w73) -> ("Error Out"=w72:errorcluster, "Background File/Folder Path"=w53:path[])  [unwired: 8 in, 1 out]
        n25 = Initialize Array(1.0 ("element"), w78) -> (w83:dbl[])
        n26 = Array Size(array=w53) -> (size(s)=w54:i32)
        n27 = Not Equal?(x=w85, y=w78) -> (x != y?=w87:bool)
        n28 = Merge Errors(w72, w57) -> (w58:errorcluster)
        n29 = Decrement(x=w54) -> (x-1=w52:i32)
        n30 = Select(t=w83, s=w87, f=w79) -> (s? t:f=w86:dbl[])
        n31 = for {
          shift-right: [w170] -> w99
          shift-left: w102 -> [w149]
          shift-right: [w168] -> w97
          shift-left: w58 -> [w150]
          tunnel: w55 -> [w166] mode=indexing
          tunnel: w75 -> [w167]
          tunnel: w80 -> [w164]
          tunnel: w89 -> [w165]
          tunnel: w86 -> [w160] mode=indexing
          tunnel: [w158] -> w74 mode=indexing
          tunnel: w56 -> [w155]
          tunnel: w53 -> [w145]
          tunnel: w52 -> [w143]
          i -> [w142]
          w152 = T11 {"FLI Dataset Type"=enum."HDF5 FLI Dataset", "No Dialog?"=TRUE, "File Path"=path ""}  # no dialog
          n32 = Build Path(base path=w167, name or relative path=w166) -> (appended path=w158:path)
          n33 = case shown="\"HDF5 FLI Dataset Series\"" w164 {
            tunnel: [_ AlliGator_FLI_Dataset_Type."Gate Image Folder" ("FLI Dataset Type") AlliGator_FLI_Dataset_Type."SS2 FLI Dataset" ("FLI Dataset Type") AlliGator_FLI_Dataset_Type.".sdt FLI Dataset (Becker & Hickl)" ("FLI Dataset Type") AlliGator_FLI_Dataset_Type.".ptu FLI Dataset (PicoQuant)" ("FLI Dataset Type") AlliGator_FLI_Dataset_Type."HDF5 FLI Dataset" ("FLI Dataset Type")] -> w162
            frame "Not a Supported Series", Default {
            }
            frame "Gate Images Folder Series" {
            }
            frame "SwissSPAD 2 Dataset Series" {
            }
            frame "B&H FLI Dataset Series" {
            }
            frame "PicoQuant PTU FLI Dataset Series" {
            }
            frame "HDF5 FLI Dataset Series" {
            }
          }
          n34 = In Range and Coerce(upper limit=w143, x=w142, lower limit=0) -> (coerced(x)=w141:i32)  [unwired: 1 out]
          n35 = Index Array(array=w145, index=w141) -> (element=w147:path)
          n36 = Empty String/Path?(string/path=w147) -> (empty?=w148:bool)
          n37 = case shown="\"HDF5 FLI Dataset\", Default" w162 {
            tunnel: [AlliGator_FLI_Dataset_Type."HDF5 FLI Dataset" ("FLI Dataset Type") AlliGator_FLI_Dataset_Type."Gate Image Folder" ("FLI Dataset Type") AlliGator_FLI_Dataset_Type.".sdt FLI Dataset (Becker & Hickl)" ("FLI Dataset Type") AlliGator_FLI_Dataset_Type.".ptu FLI Dataset (PicoQuant)" ("FLI Dataset Type") AlliGator_FLI_Dataset_Type."SS1 FLI Dataset" ("FLI Dataset Type") AlliGator_FLI_Dataset_Type."SS2 FLI Dataset" ("FLI Dataset Type") AlliGator_FLI_Dataset_Type."I/m/phi Dataset" ("FLI Dataset Type") AlliGator_FLI_Dataset_Type.".bin FLI Dataset (PicoQuant Binned)" ("FLI Dataset Type")] -> w151
            frame "HDF5 FLI Dataset", Default {
            }
            frame "Gate Image Folder" {
            }
            frame ".sdt FLI Dataset (Becker & Hickl)" {
            }
            frame ".ptu FLI Dataset (PicoQuant)" {
            }
            frame "SS1 FLI Dataset" {
            }
            frame "SS2 FLI Dataset" {
            }
            frame "I/m/phi Dataset" {
            }
            frame ".bin FLI Dataset (PicoQuant Binned)" {
            }
          }
          n38 = case shown="False" w148 {
            tunnel: w147 -> [w183 _]
            tunnel: [w182 _] -> w157
            frame False {
              n39 = Bundle By Name(cluster=T2 {"AlliGator Q Event"=enum."Files:Subtract Background File", "Data"=variant} ("Alligator Atomic Action"), "Data"=w183) -> (w182:T2)
            }
            frame True {
            }
          }
          n40 = disable-structure shown="Enabled" {
            disable-tunnel: [w172 _] -> w156
            disable-tunnel: w155 -> [w171 _]
            frame Disabled {
              n41 = Bundle By Name(cluster=T2 {"AlliGator Q Event"=enum."FLI Dataset:Channel Arithmetic", "Data"=variant} ("Alligator Atomic Action"), "Data"=w171) -> (w172:T2)
            }
            frame Enabled {
            }
          }
          n42 = Bundle By Name(cluster=w152, "FLI Dataset Type"=w151, "File Path"=w158) -> (w153:T11)
          n43 = Bundle By Name(cluster=T2 {"AlliGator Q Event"=enum."Files:Load FLI Dataset", "Data"=variant} ("Alligator Atomic Action"), "Data"=w153) -> (w159:T2)
          n44 = Bundle By Name(cluster=T2 {"AlliGator Q Event"=enum."FLI Dataset Series:Add Dataset to Accumulated Dataset", "Data"=variant} ("element"), "Data"=w160) -> (w161:T2)
          n45 = Build Array(w159, w157, w156, w161, T2 {"AlliGator Q Event"=enum."GUI:Increment Dataset Index", "Data"=variant} ("element")) -> (w169:T2[])
          n46 = call-poly "AlliGator Add Action(s) to Stack.vi"("Elements Order in Action Stack (Default: 2 BEFORE 1)"=w165, "Error In"=w150, "Alligator Queue Element 2"=w169, "Alligator Queue Element 1"=w149) -> ("Error Out"=w168:errorcluster, "Alligator Queue Element 1 (+ 2)"=w170:T2[])  [unwired: 6 in]
        }
        n47 = Bundle By Name(cluster=T2 {"AlliGator Q Event"=enum."FLI Dataset Series:Display Accumulated Dataset", "Data"=variant} ("Alligator Atomic Action"), "Data"=w76) -> (w77:T2)
        n48 = Build Array(w77, T2 {"AlliGator Q Event"=enum."Image:Image Histogram", "Data"=variant} ("element"), T2 {"AlliGator Q Event"=enum."Image:Image Contrast", "Data"=variant} ("element"), T2 {"AlliGator Q Event"=enum."Phasor Plot:Build Phasor Plot", "Data"=variant} ("element"), T2 {"AlliGator Q Event"=enum."Phasor Plot:Overlay Phasor ROI, Ratio or Map in Source Image", "Data"=variant} ("element"), T2 {"AlliGator Q Event"=enum."Phasor Plot:Highlight Image ROI in Phasor Plot", "Data"=variant} ("element")) -> (w94:T2[])
        n49 = call-poly "AlliGator Add Action(s) to Stack.vi"("Elements Order in Action Stack (Default: 2 BEFORE 1)"=w89, "Error In"=w97, "Alligator Queue Element 2"=w94, "Alligator Queue Element 1"=w99) -> ("Error Out"=w96:errorcluster, "Alligator Queue Element 1 (+ 2)"=w98:T2[])  [unwired: 6 in]
      }
      frame "End Script" {
        n50 = call "Current Date & Time String (High Precision).vi"() -> ("time string"=w197:string, "date string"=w194:string)  [unwired: 8 in, 2 out]
        n51 = call-poly "AlliGator Add Action(s) to Stack.vi"("Elements Order in Action Stack (Default: 2 BEFORE 1)"=Alligator_Elements_Order_in_Action_Stack."Enqueue 2 AFTER 1", "Error In"=w201, "Alligator Atomic Action"=T2 {"AlliGator Q Event"=enum."GUI:End Script", "Data"=variant} ("element"), "Alligator Queue Element 1"=w202) -> ("Error Out"=w191:errorcluster, "Alligator Queue Element 1 (+ 2)"=w199:T2[])  [unwired: 6 in]
        n52 = Format Into String(format string="Sum All Datasets in Time Series %s started on %s at %s" ("initial string"), error in=w191, w193, w194, w197) -> (resulting string=w192:string, error out=w190:errorcluster)  [unwired: 1 in]
      }
    }
    n53 = Increment(x=w28) -> (x+1=w27:T5)
  }
  "Alligator Queue Elements out" <- w12
  "# Time Points" <- w5
  "[Time-Series Path]" <- w2
  "Message" <- w1
  n54 = call "Alligator Variables Storage.vi"("Get(F)/Set"=TRUE, "AlliGator Variable"=AlliGator_Variables_List."Script in progress" ("Alligator Variable"), "Error In"=w11, "Data in"=TRUE) -> ("Error Out"=→"Error Out":errorcluster)  [unwired: 5 in, 2 out]
